vi "Read Sender.vi"(8 "error in (no error)":errorcluster, 11 "iMessage in":refnum<class "iMessage.lvclass">) -> (0 "error out":errorcluster, 2 "Sender":string, 3 "iMessage out":refnum<class "iMessage.lvclass">)   [LabVIEW 2017, in "Message Interface.lvlib" / "iMessage.lvclass"]
uses:
  iMessage.lvclass
  iMessage.lvclass/iMessage.ctl
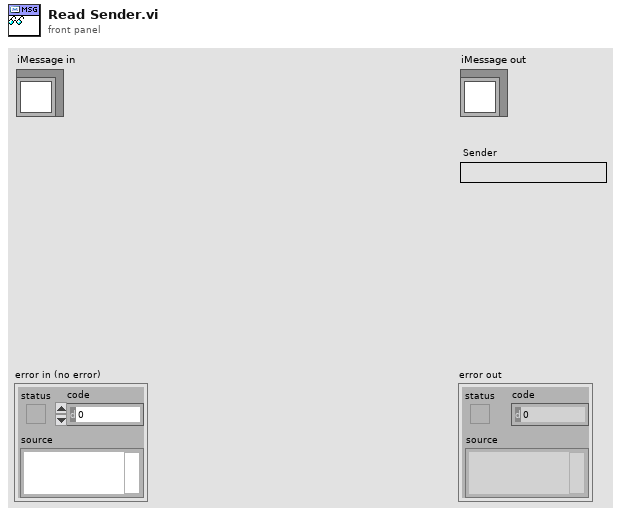
[diagram p1: front panel]
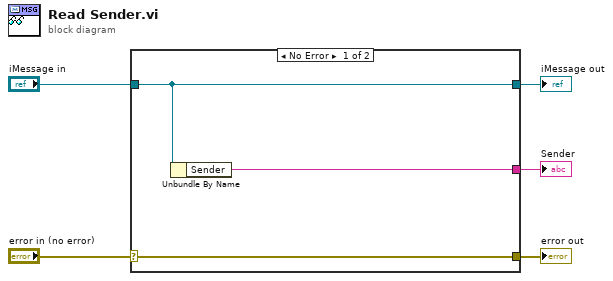
[diagram p0: block diagram]
diagram:
  n1 = case shown="No Error" "error in (no error)" {
    selector: "error in (no error)" -> [w8 w9]
    tunnel: [w8 w9] -> w4
    tunnel: [w7 w10] -> w2
    tunnel: "iMessage in" -> [w7 w10]
    tunnel: [w6 _] -> w1
    frame No Error {
      n2 = Unbundle By Name(w7) -> ("Sender"=w6:string)
    }
    frame Error {
    }
  }
  "error out" <- w4
  "iMessage out" <- w2
  "Sender" <- w1
